vi "Pick Up Order.vi"(8 "error in (no error)":errorcluster, 10 "Worker":refnum<class "Beverage.lvclass">, 11 "Mock Worker Processor In":refnum<class "Mock Pick Up Order.lvclass">) -> (0 "error out":errorcluster, 3 "Mock Worker Processor Out":refnum<class "Mock Pick Up Order.lvclass">)   [LabVIEW 2020, in "Mock Pick Up Order.lvclass"]
uses:
  Mock Pick Up Order.lvclass
  Support/Beverages/Beverage/Beverage.lvclass
  Mock Pick Up Order.lvclass/Mock Pick Up Order.ctl
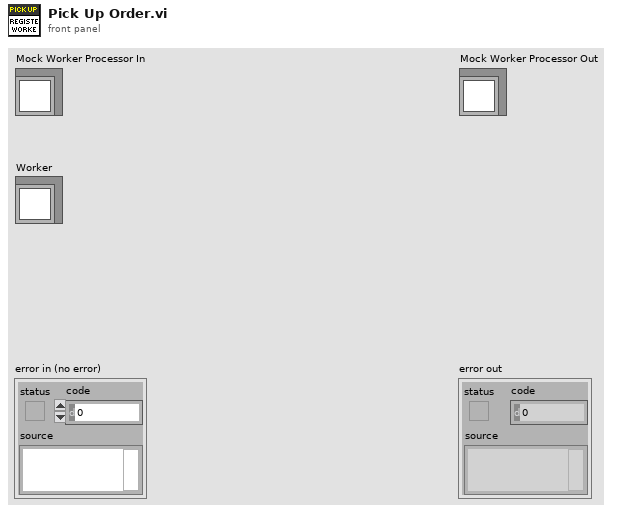
[diagram p1: front panel]
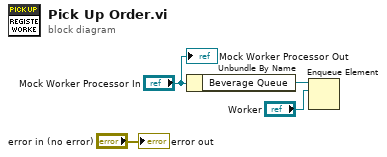
[diagram p0: block diagram]
diagram:
  n1 = Unbundle By Name("Mock Worker Processor In") -> ("Beverage Queue"=w3:refnum<queue>)
  n2 = Enqueue Element(queue=w3, element="Worker") -> ()  [unwired: 2 in, 3 out]
  "error out" <- "error in (no error)"
  "Mock Worker Processor Out" <- "Mock Worker Processor In"
